vi "ExposeDestroy.vi"(8 "error in (no error)":errorcluster, 11 "Expose Info":T1) -> (0 "error out":errorcluster, 3 "Expose Info out":T1)   [LabVIEW 2017]
uses:
  ExposeInfo.ctl
  C:/Code/CMCryoSysCode/Expose/COM/CSCom/CSCom/bin/Release/CSCom.dll
  COM/CSCom/CSCom/bin/Release/CSCom.dll
  ExposeMessage.ctl
  Events/ExposeMessageType.ctl
  Mapper/ExposeObjectMapNamepathData.ctl
  Mapper/ExposeMapperDataTypeEnum.ctl
  Mapper/ExposeObjectMapContainerTypeEnum.ctl
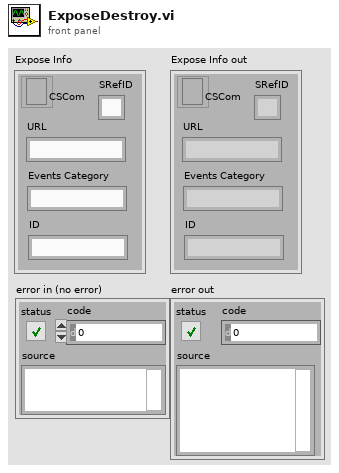
[diagram p1: front panel]
types:
  T1 = typedef "ExposeInfo.ctl" = cluster{"CSCom":refnum<k24>, "URL":string, "Events Category":string, "ID":string, "SRefID":string}
  T2 = typedef "ExposeMessage.ctl" = cluster{"Message Type":T3, "Text":string, "NamepathInfo":T4[]}
  T3 = typedef "ExposeMessageType.ctl" = i32
  T4 = typedef "ExposeObjectMapNamepathData.ctl" = cluster{"Type":T5, "Value":variant, "Namepath":string, "Container Type":T6}
  T5 = typedef "ExposeMapperDataTypeEnum.ctl" = enum16{"NotData", "int8", "byte", "int16", "uint16", "int32", "uint32", "int64", "uint64", "Single", "Double", "String", "Boolean", "Container"}
  T6 = typedef "ExposeObjectMapContainerTypeEnum.ctl" = enum16{"Value", "Array", "Waveform", "NetContainer"}
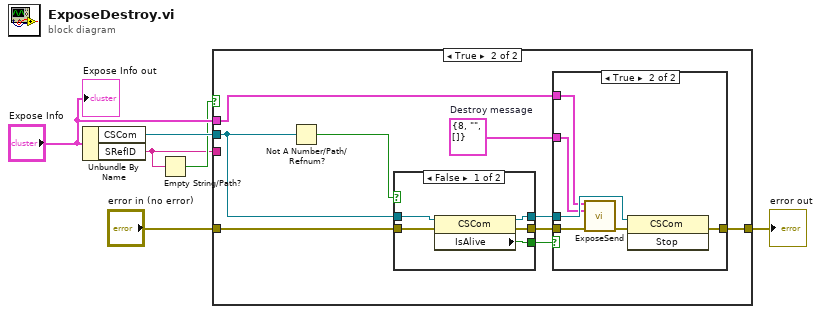
[diagram p0: block diagram]
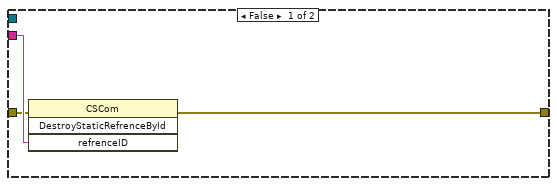
[diagram p2: hidden frame]
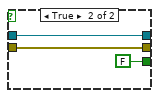
[diagram p3: hidden frame]
diagram:
  n1 = Unbundle By Name("Expose Info") -> ("CSCom"=w3:refnum<k24>, "SRefID"=w1:string)
  n2 = Empty String/Path?(string/path=w1) -> (empty?=w2:bool)
  n3 = case shown="True" w2 {
    tunnel: [w7 w18] -> w6
    tunnel: "Expose Info" -> [_ w16]
    tunnel: "error in (no error)" -> [w8 w13]
    tunnel: w3 -> [_ w11]
    tunnel: w1 -> [w9 _]
    frame False {
      n4 = invoke class="CSCom" method="DestroyStaticRefrenceById"(error in=w8, "refrenceID"=w9) -> (error out=w7:errorcluster)  [unwired: 2 in, 3 out]
    }
    frame True {
      w15 = T2 {"Message Type"=8, "Text"="", "NamepathInfo"=[]}  # Destroy message
      n5 = Not A Number/Path/Refnum?(number/path/refnum=w11) -> (NaN/Path/Refnum?=w10:bool)
      n6 = case shown="False" w10 {
        tunnel: [w23 w24] -> w17
        tunnel: [w22 w25] -> w14
        tunnel: w13 -> [w21 w25]
        tunnel: [w20 FALSE ("IsAlive")] -> w12
        tunnel: w11 -> [w19 w24]
        frame False {
          n7 = property class="CSCom"(reference=w19, error in=w21) -> (reference out=w23:refnum<k24>, error out=w22:errorcluster, "IsAlive"=w20:bool)
        }
        frame True {
        }
      }
      n8 = case shown="True" w12 {
        tunnel: [w27 w33] -> w18
        tunnel: w17 -> [_ w32]
        tunnel: w16 -> [_ w31]
        tunnel: w15 -> [_ w30]
        tunnel: w14 -> [w27 w29]
        frame False {
        }
        frame True {
          n9 = call "ExposeSend.vi"("Expose"=w31, "Message"=w30, "error in (no error)"=w29) -> ("error out"=w28:errorcluster)  [unwired: 10 in, 2 out]
          n10 = invoke class="CSCom" method="Stop"(reference=w32, error in=w28) -> (error out=w33:errorcluster)  [unwired: 1 in, 2 out]
        }
      }
    }
  }
  "error out" <- w6
  "Expose Info out" <- "Expose Info"
